vi "LoadControlPanel.vi"(8 "error in (no error)":errorcluster, 10 "Actor In":refnum<class "Actor.lvclass">, 11 "GRMActor in":refnum<class "FlatField.lvclass">) -> (0 "error out":errorcluster, 3 "GRMActor out":refnum<class "FlatField.lvclass">)   [LabVIEW 2020, in "FlatField.lvlib" / "FlatField.lvclass"]
uses:
  FlatField.lvclass
  <vilib>/ActorFramework/Actor/Actor.lvclass
  FlatFieldUI/FlatFieldUI.lvclass
  C:/Program Files/National Instruments/LabVIEW 2020/vi.lib/ActorFramework/Actor/Actor.lvclass
  Model/Hardware Abstraction Layer/Component/GenericActor/GenericActor/GenericActor.lvclass
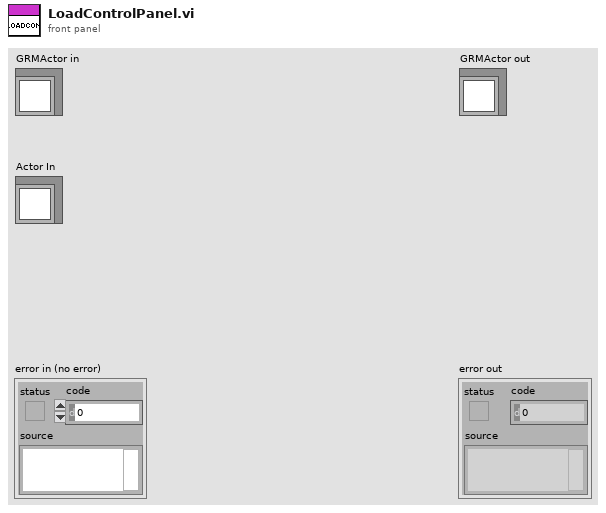
[diagram p1: front panel]
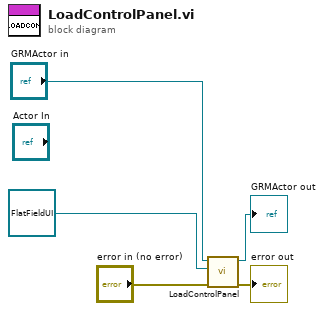
[diagram p0: block diagram]
diagram:
  n1 = call-parent "LoadControlPanel.vi"("error in (no error)"="error in (no error)", "Actor In"=refnum<class "FlatFieldUI.lvclass"> refnum ("FlatField.lvlib:FlatFieldUI.lvlib:FlatFieldUI.lvclass"), "GRMActor in"="GRMActor in") -> ("error out"=→"error out":errorcluster, "GRMActor out"=→"GRMActor out":refnum<class "FlatField.lvclass">)  [unwired: 7 in]
